vi "RunMyNewModuleInPEF.vi"(3 "error in (no error)":errorcluster) -> (10 "error out":errorcluster)   [LabVIEW 2020]
uses:
  <vilib>/ADAS Record/PEFInterface/subVIs/NI.Pef.Interface.lvclass
  <vilib>/ADAS Record/Utilities/ADAS Utilities.lvlib
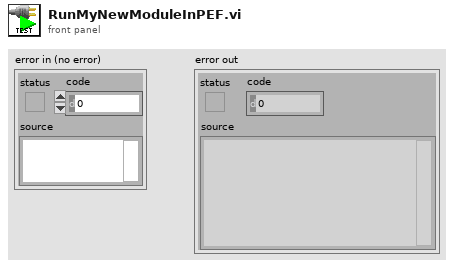
[diagram p1: front panel]
types:
  T1 = typedef "ADAS Utilities.lvlib/System Config.ctl" = cluster{"Description":string, "Version":T2, "IO Plugins":T3[], "IO Links":T4[], "UI Plugins":T6[], "Layout Links":T7[]}
  T2 = typedef "ADAS Utilities.lvlib/Config Version.ctl" = cluster{"Major":u32, "Minor":u32, "Fix":u32, "Build":u32}
  T3 = typedef "ADAS Utilities.lvlib/IO Plugin Instance.ctl" = cluster{"Type ID":string, "Instance ID":string, "Config String":string, "Display Name":string, "Description":string}
  T4 = typedef "ADAS Utilities.lvlib/Link.ctl" = cluster{"Source":T5, "Destination":T5}
  T5 = typedef "ADAS Utilities.lvlib/Stream.ctl" = cluster{"Instance ID":string, "Terminal":string}
  T6 = typedef "ADAS Utilities.lvlib/UI Plugin Instance.ctl" = cluster{"Type ID":string, "Instance ID":string, "Display Name":string, "Description":string, "Common Config String":string, "Custom Config String":string}
  T7 = typedef "ADAS Utilities.lvlib/Layout Link.ctl" = cluster{"Plugin Instance ID":string, "Cell Descriptor":string, "Cell Display Name":string}
  T8 = typedef "NI.Pef.Interface.lvlib/NI.Pef.Interface.lvclass/PEF Interface - PE Info.ctl" = cluster{"Alias":string, "Output Terminal Names":string[]}
  T9 = cluster{"Data Producer":T8, "Data Producer Output Terminal Index":u32, "Data Consumer":T8}[]
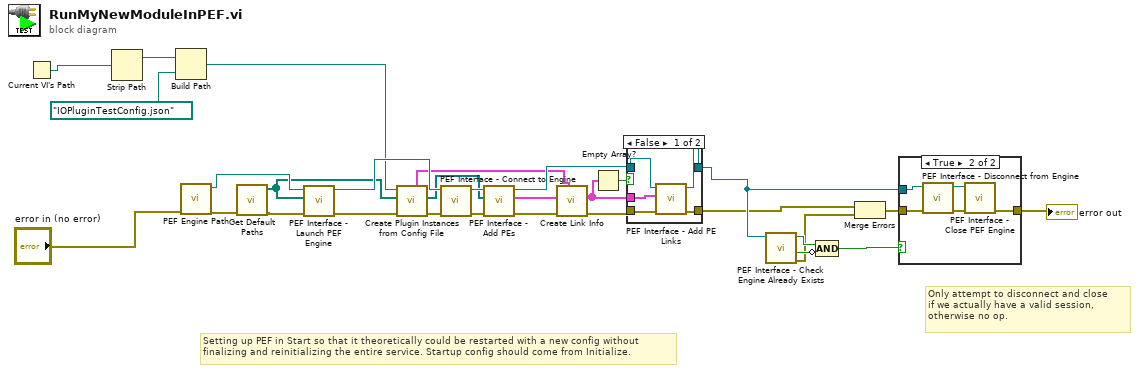
[diagram p0: block diagram]
diagram:
  # "Only attempt to disconnect and close \nif we actually have a valid session, \notherwise no op."
  # "Setting up PEF in Start so that it theoretically could be restarted with a new config without\nfinalizing and reinitializing the entire service. Startup config should come from Initialize."
  n1 = Current VI's Path() -> (path=w21:path)
  n2 = Strip Path(path=w21) -> (stripped path=w20:path)  [unwired: 1 out]
  n3 = Build Path(base path=w20, name or relative path=path "IOPluginTestConfig.json") -> (appended path=w12:path)
  n4 = call <vilib>:"PEF Engine Path.vi"("error in (no error)"="error in (no error)") -> ("error out"=w16:errorcluster, "appended path"=w17:path)  [unwired: 9 in]
  n5 = call <vilib>:"Get Default Paths.vi"("error in (no error)"=w16) -> ("error out"=w18:errorcluster, "Default IO Plugin Directories"=w13:path[])  [unwired: 6 in, 3 out]
  n6 = call <vilib>:"PEF Interface - Launch PEF Engine.vi"("error in (no error)"=w18, "User Plugin Folders"=w13, "PEF Engine Path (Newest Installed)"=w17) -> ("error out"=w15:errorcluster, "PEF Session Out"=w27:refnum<class "NI.Pef.Interface.lvclass">)  [unwired: 7 in]
  n7 = call <vilib>:"Create Plugin Instances from Config File.vi"("error in (no error)"=w15, "IO plugin directories"=w13, "sys config file path"=w12) -> ("error out"=w14:errorcluster, "Plugin Instances to Add"=w11:refnum<class "Processing Element Specification.lvclass">[], "System Config"=w8:T1)  [unwired: 6 in]
  n8 = call <vilib>:"PEF Interface - Connect to Engine.vi"("error in (no error)"=w14, "PEF Session In (Optional)"=w27) -> ("error out"=w29:errorcluster, "PEF Session Out"=w28:refnum<class "NI.Pef.Interface.lvclass">)  [unwired: 7 in, 1 out]
  n9 = call <vilib>:"PEF Interface - Add PEs.vi"("error in (no error)"=w29, "PE References to Add"=w11, "PEF Session In"=w28) -> ("error out"=w10:errorcluster, "PE Info"=w9:T8[], "PEF Session Out"=w30:refnum<class "NI.Pef.Interface.lvclass">)  [unwired: 5 in, 1 out]
  n10 = call <vilib>:"Create Link Info.vi"("System Config In"=w8, "error in (no error)"=w10, "PEF: PE Info In"=w9) -> ("error out"=w6:errorcluster, "PEF: Link Arrray Out"=w7:T9)  [unwired: 7 in]
  n11 = Empty Array?(array=w7) -> (empty?=w26:bool)
  n12 = case shown="False" w26 {
    tunnel: w7 -> [w35 _]
    tunnel: w6 -> [w34 w36]
    tunnel: w30 -> [w33 w37]
    tunnel: [w32 w37] -> w22
    tunnel: [w31 w36] -> w2
    frame False {
      n13 = call <vilib>:"PEF Interface - Add PE Links.vi"("error in (no error)"=w34, "PE Links"=w35, "PEF Session In"=w33) -> ("error out"=w31:errorcluster, "PEF Session Out"=w32:refnum<class "NI.Pef.Interface.lvclass">)  [unwired: 6 in, 1 out]
    }
    frame True {
    }
  }
  n14 = call <vilib>:"PEF Interface - Check Engine Already Exists.vi"("PEF Session In"=w22) -> ("error out"=w3:errorcluster, "Empty Session"=w24:bool, "PEF/FlexLogger Open"=w25:bool)  [unwired: 7 in, 1 out]
  n15 = Compound Arithmetic op=AND(w25, invert w24) -> (w23:bool)
  n16 = Merge Errors(w2, w3) -> (w1:errorcluster)
  n17 = case shown="True" w23 {
    tunnel: w1 -> [w38 w42]
    tunnel: [w38 w41] -> w4
    tunnel: w22 -> [_ w39]
    frame False {
    }
    frame True {
      n18 = call <vilib>:"PEF Interface - Disconnect from Engine.vi"("error in (no error)"=w42, "PEF Session In"=w39) -> ("error out"=w43:errorcluster, "PEF Session Out"=w40:refnum<class "NI.Pef.Interface.lvclass">)  [unwired: 8 in]
      n19 = call <vilib>:"PEF Interface - Close PEF Engine.vi"("error in (no error)"=w43, "PEF Session In"=w40) -> ("error out"=w41:errorcluster)  [unwired: 9 in]
    }
  }
  "error out" <- w4
